vi "Test_GetUninstall.vi"(3 "error in":errorcluster, 5 "Break":refnum<k21>) -> (0 "error out":errorcluster, 1 "unIndex":bool[](array[boolean]), 2 "numUninstall":i32)   [LabVIEW 2015]
doc: "测试前判断工位是否安装了断路器\nunIndex\n安装的=0\n未安装的=-1"
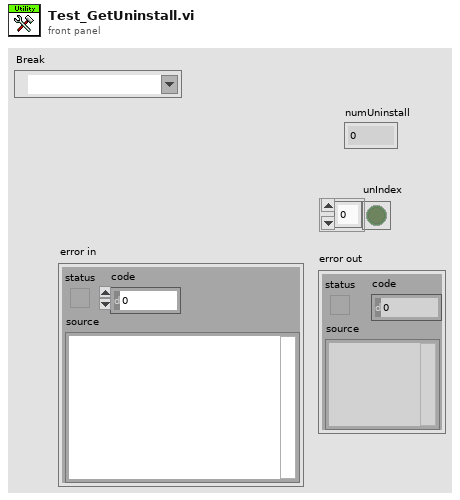
[diagram p1: front panel]
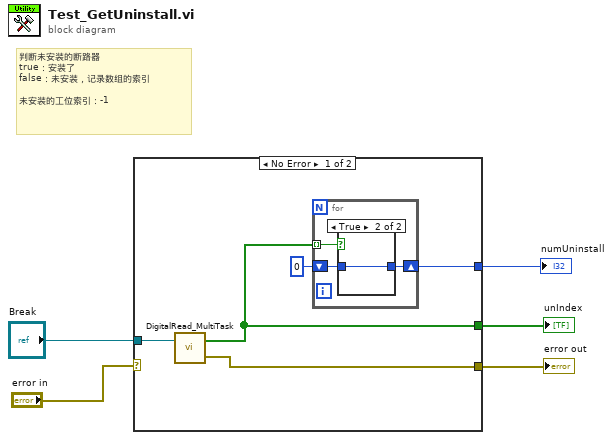
[diagram p0: block diagram]
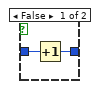
[diagram p2: hidden frame]
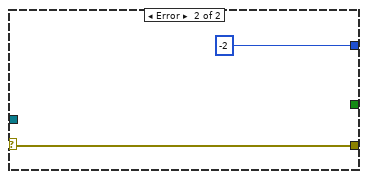
[diagram p3: hidden frame]
diagram:
  # "判断未安装的断路器\ntrue：安装了\nfalse：未安装，记录数组的索引\n\n未安装的工位索引：-1"
  n1 = case shown="No Error" "error in" {
    selector: "error in" -> [_ w17]
    tunnel: "Break" -> [w7 _]
    tunnel: [w6 w17] -> w4
    tunnel: [w9 -2] -> w3
    tunnel: [w8 _] -> w1
    frame No Error {
      n2 = call "DigitalRead_MultiTask.vi"("mutiTask"=w7) -> ("error out"=w6:errorcluster, "read"=w8:bool[])  [unwired: 1 in]
      n3 = for {
        tunnel: w8 -> [w13] mode=indexing
        shift-right: [w12] -> w9
        shift-left: 0 -> [w11]
        n4 = case shown="True" w13 {
          tunnel: [w15 w16] -> w12
          tunnel: w11 -> [w14 w16]
          frame False {
            n5 = Increment(x=w14) -> (x+1=w15:i32)
          }
          frame True {
          }
        }
      }
    }
    frame Error {
    }
  }
  "error out" <- w4
  "numUninstall" <- w3
  "unIndex" <- w1
